vi "Track Goals.vi"(10 "Goal Display":T2(plugin-control), 11 "Original Image":T2(plugin-control)) -> (2 "Traget Line Mask Out":T2(plugin-control), 3 "Goal Display Out":T2(plugin-control))   [LabVIEW 2016]
uses:
  Camera Types.ctl
panel:
  in  "Camera Type":T1=enum."1013"
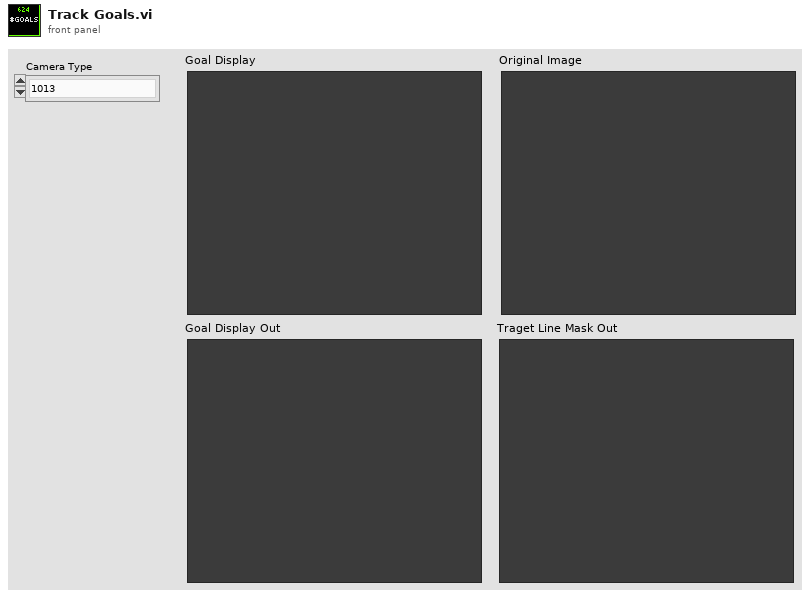
[diagram p1: front panel]
types:
  T1 = typedef "Camera Types.ctl" = enum16{"206", "1011", "1013", "MS HD3000 square", "MS HD3000 640x480"}
  T2 = typedef "IMAQ Image.ctl" = refnum<image>
  T3 = cluster{"Distance (ft)":dbl, "Score":dbl, "Normalized":cluster{"Center":cluster{dbl, dbl}, "Rectangle":cluster{"Numeric":dbl, "Numeric 2":dbl, "Numeric 3":dbl, "Numeric 5":dbl}}, "Pixels":cluster{"Center":cluster{dbl, dbl}, "Rectangle":cluster{"Numeric":dbl, "Numeric 2":dbl, "Numeric 3":dbl, "Numeric 5":dbl}}}
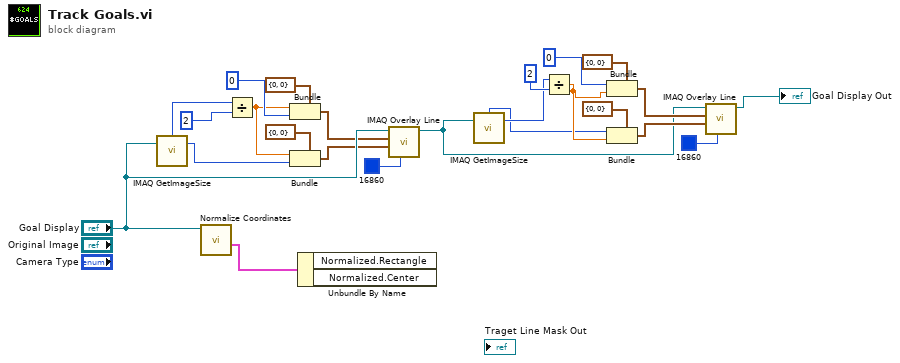
[diagram p0: block diagram]
diagram:
  n1 = call "IMAQ GetImageSize"("Image"="Goal Display") -> ("Y Resolution"=w19:i32, "X Resolution"=w24:i32)  [unwired: 3 in, 1 out]
  n2 = call "Normalize Coordinates.vi"("Image in"="Goal Display") -> ("Results"=w1:T3)  [unwired: 9 in, 1 out]
  n3 = Divide(x=w24, y=2) -> (x/y=w18:dbl)
  n4 = Bundle(cluster=cluster{"X":i32, "Y":i32} {"X"=0, "Y"=0} ("Start Point"), "X"=w18, "Y"=0) -> (w15:cluster{"X":i32, "Y":i32})
  n5 = Bundle(cluster=cluster{"X":i32, "Y":i32} {"X"=0, "Y"=0} ("Start Point"), "X"=w18, "Y"=w19) -> (w16:cluster{"X":i32, "Y":i32})
  n6 = Unbundle By Name(w1) -> ()  [unwired: 2 out]
  n7 = call "IMAQ Overlay Line"("Color"=u32 16860, "End Point"=w16, "Start Point"=w15, "Image"="Goal Display") -> ("Image Out"=w7:T2)  [unwired: 6 in, 1 out]
  n8 = call "IMAQ GetImageSize"("Image"=w7) -> ("Y Resolution"=w6:i32, "X Resolution"=w3:i32)  [unwired: 3 in, 1 out]
  n9 = Divide(x=w6, y=2) -> (x/y=w4:dbl)
  n10 = Bundle(cluster=cluster{"X":i32, "Y":i32} {"X"=0, "Y"=0} ("Start Point"), "X"=0 ("Y"), "Y"=w4) -> (w12:cluster{"X":i32, "Y":i32})
  n11 = Bundle(cluster=cluster{"X":i32, "Y":i32} {"X"=0, "Y"=0} ("Start Point"), "X"=w3, "Y"=w4) -> (w11:cluster{"X":i32, "Y":i32})
  n12 = call "IMAQ Overlay Line"("Color"=u32 16860, "End Point"=w11, "Start Point"=w12, "Image"=w7) -> ("Image Out"=→"Goal Display Out":T2)  [unwired: 6 in, 1 out]
